vi "Actor Core.vi"(8 "error in":errorcluster, 11 "Proxy in":refnum<class "Proxy.lvclass">) -> (0 "error out":errorcluster, 3 "Actor out":refnum<class "Actor.lvclass">)   [LabVIEW 2014, in "Proxy.lvlib" / "Proxy.lvclass"]
doc: "(<B>Filename</B>: Actor Framework.lvlib:Actor.lvclass:Actor Core.vi)\n\nReceives messages to the actor, reacts to them, and initiates any error handling that may shut the actor down.\n\nDescendant classes may override this VI to append parallel tasks for the actor to complete while it handles messages. Overrides use the Call Parent Method node."
uses:
  Proxy.lvclass
  <vilib>/ActorFramework/Actor/Actor.lvclass
  Target/Target/Target.lvclass
  Proxy.lvclass/Proxy.ctl
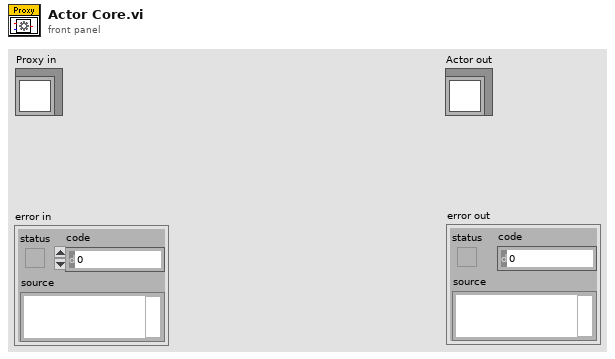
[diagram p1: front panel]
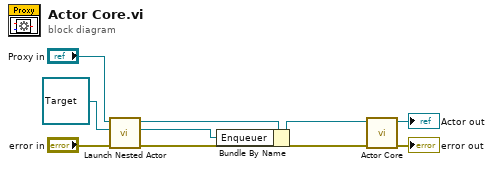
[diagram p0: block diagram]
diagram:
  n1 = call <vilib>:"Launch Nested Actor.vi"("error in (no error)"="error in", "Nested Actor"=refnum<class "Target.lvclass"> refnum ("Target.lvlib:Target.lvclass"), "Caller Actor in"="Proxy in") -> ("error out"=w3:errorcluster, "Nested Actor's Enqueuer"=w1:refnum<class "Message Enqueuer.lvclass">, "Caller Actor out"=w6:refnum<class "Proxy.lvclass">)  [unwired: 6 in]
  n2 = Bundle By Name(cluster=w6, "Enqueuer"=w1) -> (w2:refnum<class "Proxy.lvclass">)
  n3 = call-parent "Actor Core.vi"("error in"=w3, "Actor in"=w2) -> ("error out"=→"error out":errorcluster, "Actor out"=→"Actor out":refnum<class "Actor.lvclass">)  [unwired: 8 in]
